vi "sequence utility.vi"(7 "sequence in":string[](array[string]), 8 "error in (no error)":errorcluster, 9 "sequence path":path=path "C:/Users/shared/Sequences/MPMS_LCR_Tsweep.vi.txt", 10 "platform":u16(ring)=1 items=["Mac", "PC"], 11 "export?":bool) -> (0 "error out":errorcluster, 2 "changed sequence":string[](array[string]), 3 "do not update seq.":bool)   [LabVIEW 2024]
doc: "Sequence Program with the Message Handling Queue (MHQ) for the National High Magnetic Field Laboratory in Tallahassee, Florida. \nOnce you understand how the programs works, you should be able to modify this program easily. If you have any questions, contact Minseong Lee(ml10k@my.fsu.edu), who first made this program in June, 2015."
panel:
  in  "edit":bool
  in  "audit":bool
  in  "accept/return":bool
  in  "Loop":bool
  in  "Replace":bool
  in  "cancel":bool
  out "Buffer Edit":string[](array[string])=["Wait for 1 s", "Wait for 2 s", "Wait for 1.1 s", "Wait for 1.2 s"]
  out "Path":path=path "C:/Users/shared/Sequences/MPMS_LCR_Tsweep.vi.txt"
  out "Buffer History":string[](array[string])
  in  "New Button":bool caption="New"
  in  "Commands":string(tree)="Wait for"
  in  "Sequence":i32[](listbox)=[4]
  in  "Save Button":bool caption="Save"
  in  "Save As Button":bool caption="Save As"
  out "Cursor Position":i32=4
  in  "Open Button":bool caption="Open"
  # "Sequence Editor"
  # "changes to the main monovu.vi"
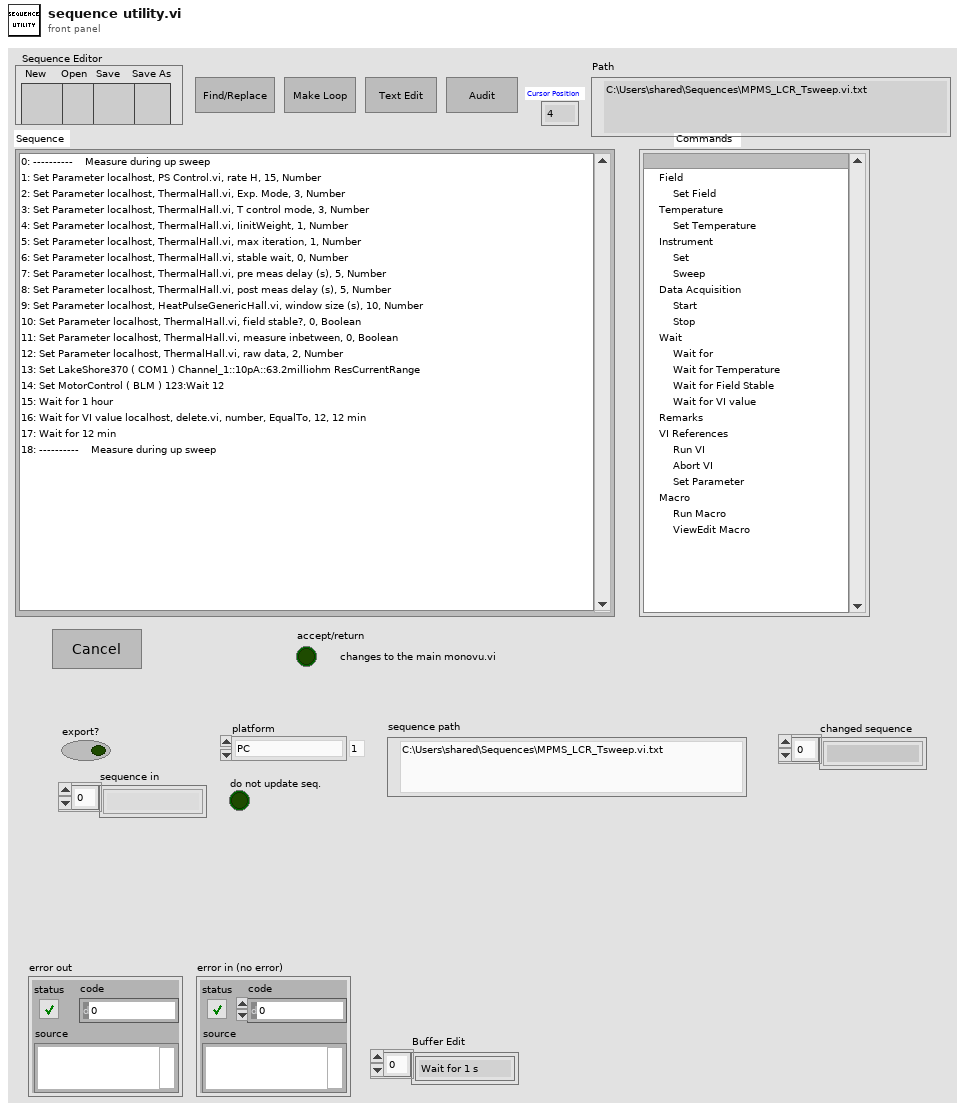
[diagram p1: front panel]
types:
  T1 = cluster{"No. of command":i32, "Parameters":string[], "Address":refnum<visa-resource-name>, "Boolean":bool, "No. of line":i32, "Initial Time":timestamp, "Current Time":timestamp, "Sequence status":string, "Sequence":refnum<vi>, "Temp_Check":i32, "Sequence_History":string, "Subsequence":string[]}
  T2 = cluster{"number of line":i32, "Signal":bool, "Command":string, "Sequence Reference":refnum<vi>, "Add or modification":bool}
  T3 = typedef "Command_Message.ctl" = cluster{"No. of command":i32, "Parameters":string[], "Address":refnum<visa-resource-name>, "Boolean":bool, "No. of line":i32, "Initial Time":timestamp, "Current Time":timestamp, "Status":string, "Sequence Ref.":refnum<vi>, "Temp check":i32, "Sequence_History":string, "Subsequence":string[]}
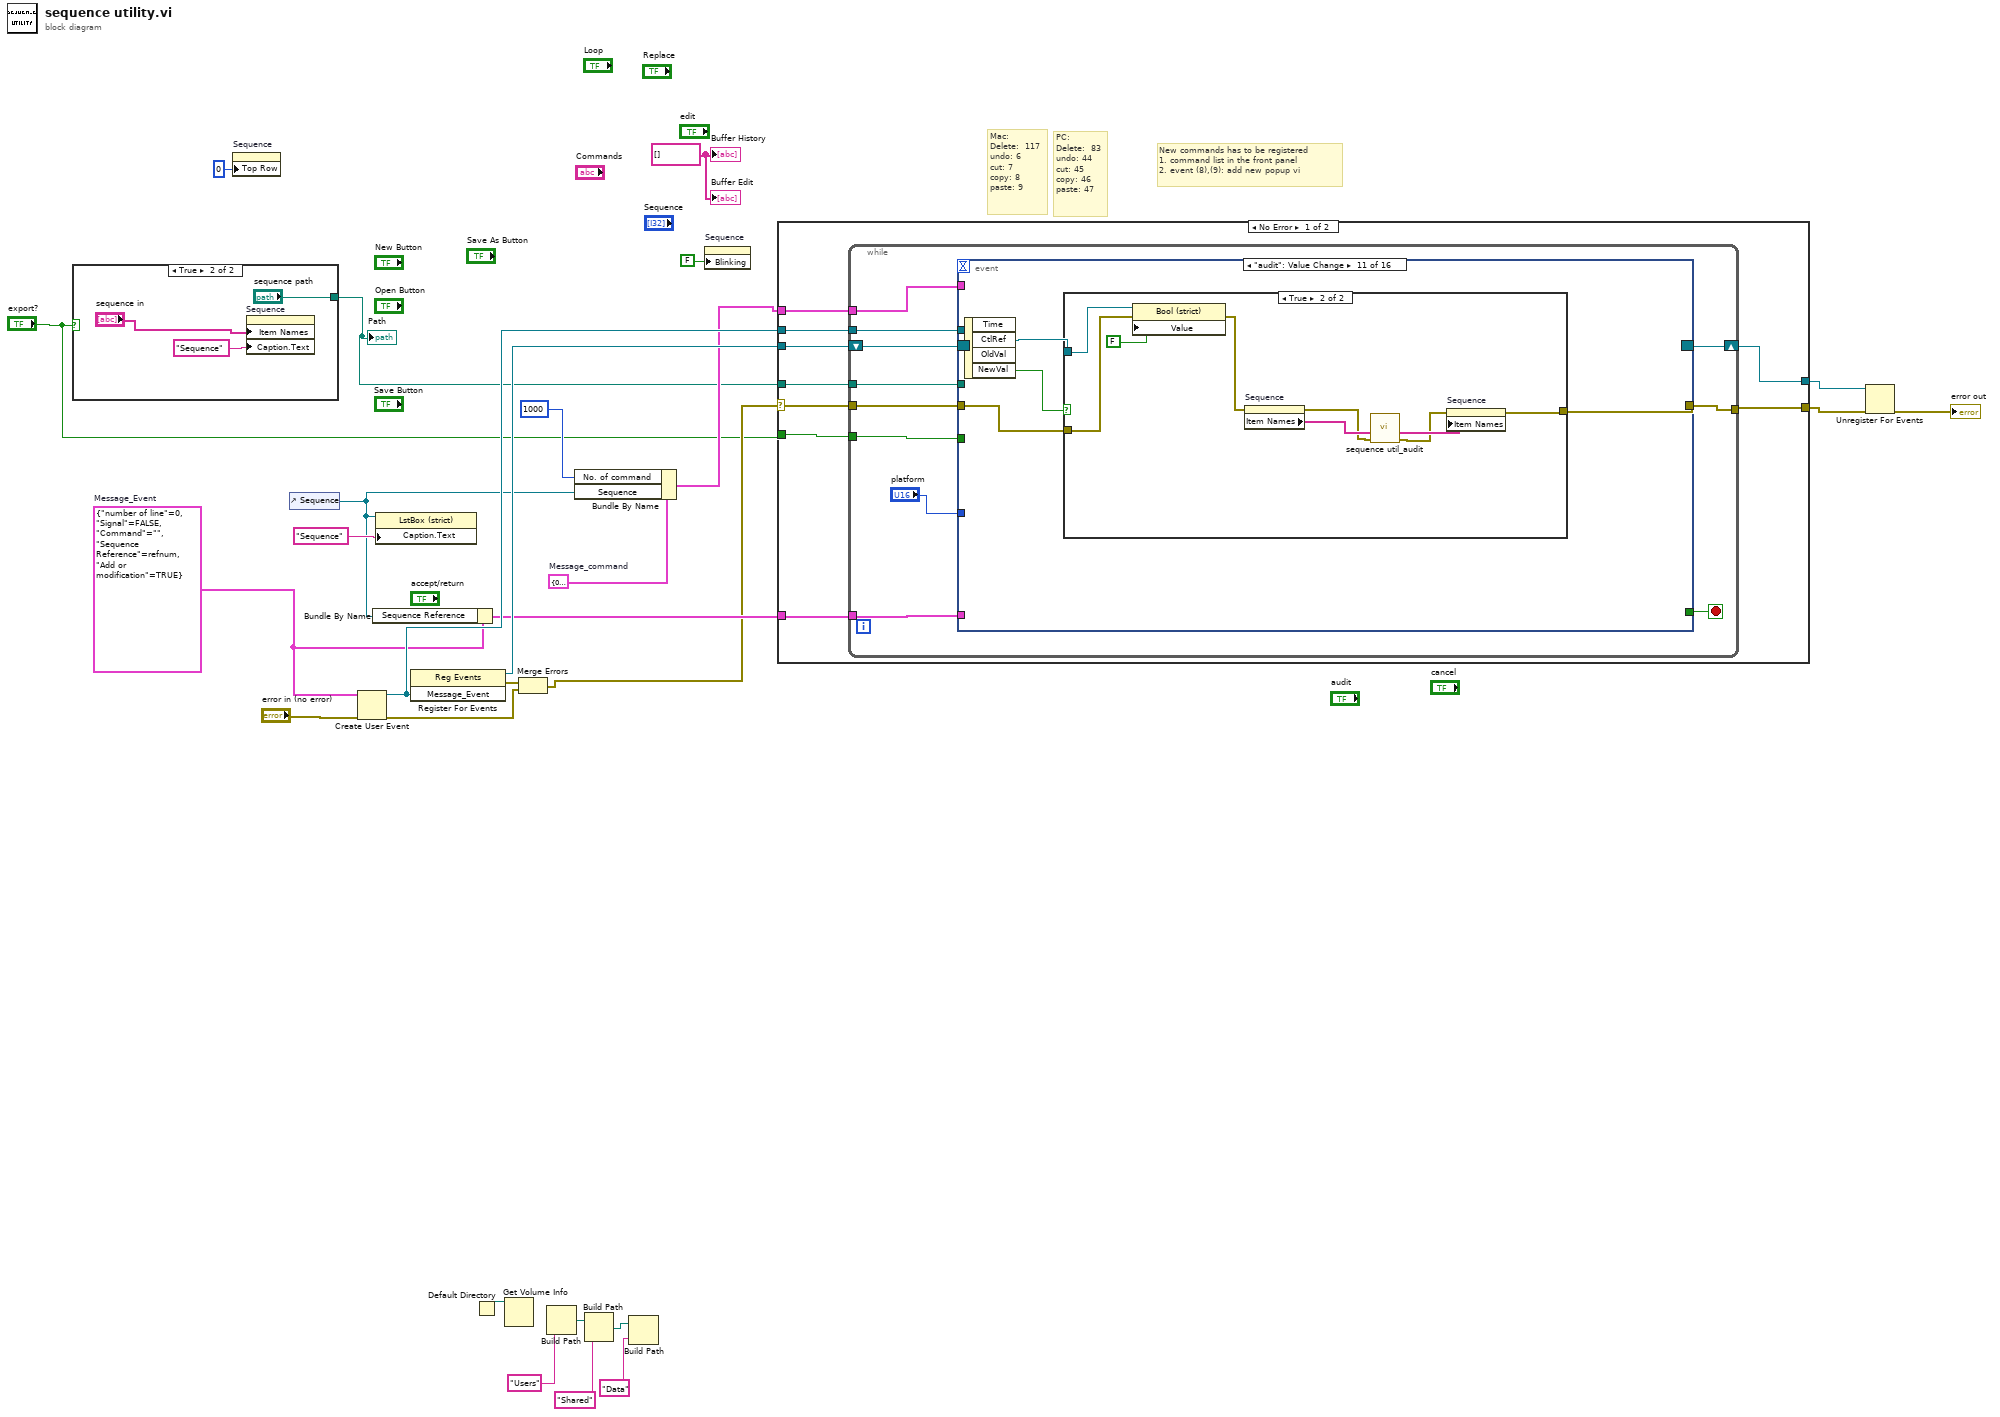
[diagram p0: block diagram]
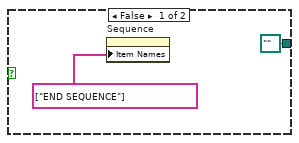
[diagram p2: hidden frame]
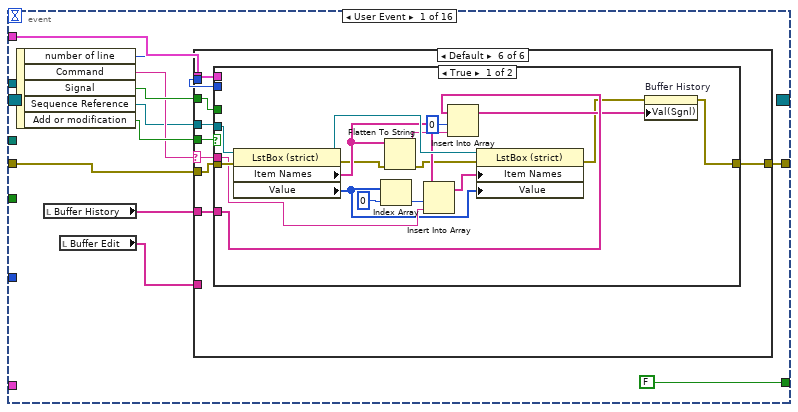
[diagram p3: hidden frame]
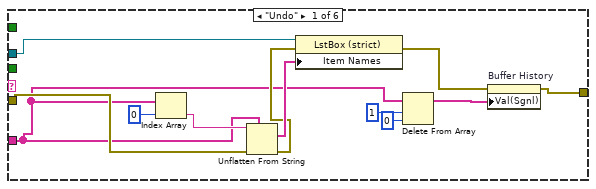
[diagram p4: hidden frame]
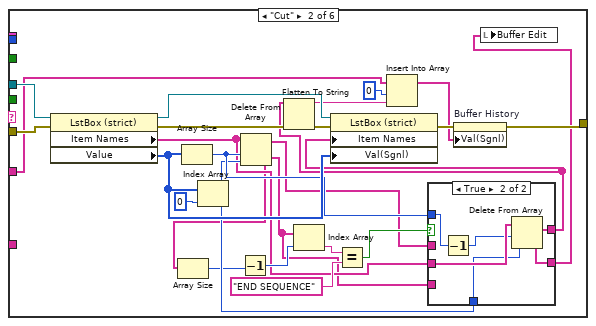
[diagram p5: hidden frame]
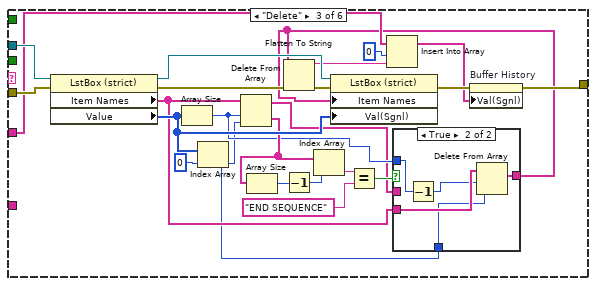
[diagram p7: hidden frame]
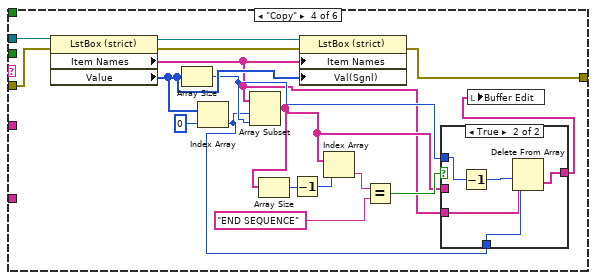
[diagram p9: hidden frame]
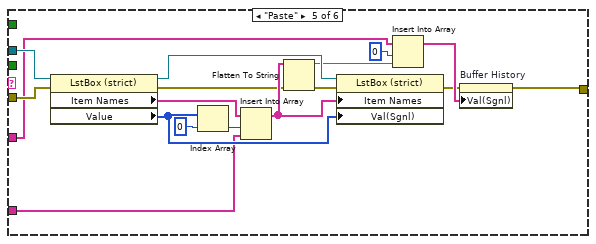
[diagram p11: hidden frame]
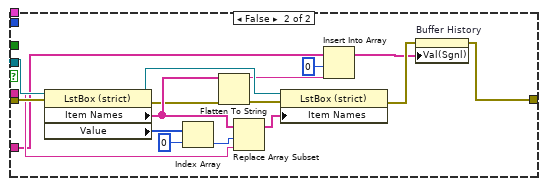
[diagram p12: hidden frame]
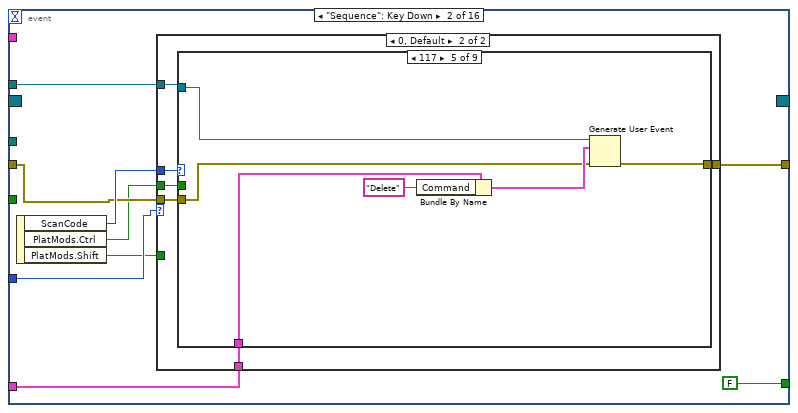
[diagram p13: hidden frame]
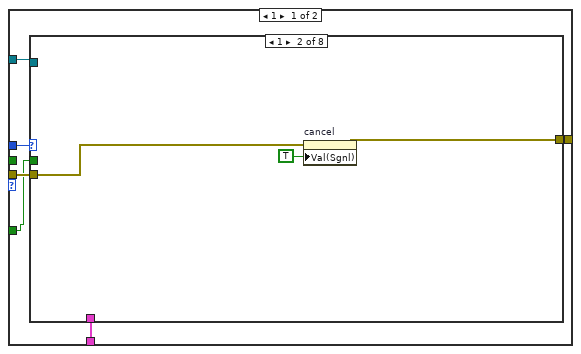
[diagram p14: hidden frame]
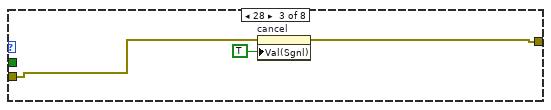
[diagram p16: hidden frame]
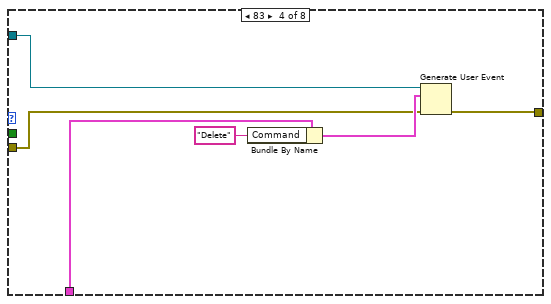
[diagram p17: hidden frame]
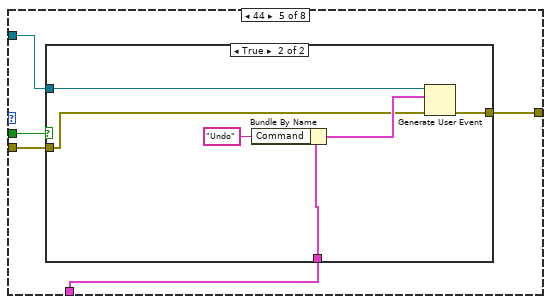
[diagram p18: hidden frame]
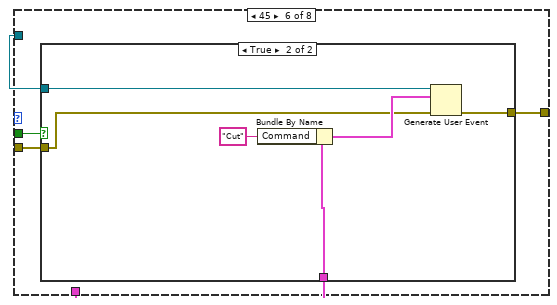
[diagram p20: hidden frame]
diagram:
  w5 = T1 {"No. of command"=0, "Parameters"=[], "Address"="", "Boolean"=TRUE, "No. of line"=0, "Initial Time"=timestamp(0 s since 1904-01-01), "Current Time"=timestamp(0 s since 1904-01-01), "Sequence status"="", "Sequence"=refnum, "Temp_Check"=0, "Sequence_History"="", "Subsequence"=[]}  # Message_command
  w15 = string[] []
  w20 = T2 {"number of line"=0, "Signal"=FALSE, "Command"="", "Sequence Reference"=refnum, "Add or modification"=TRUE}  # Message_Event
  # "New commands has to be registered\n1. command list in the front panel\n2. event (8),(9): add new popup vi"
  # "PC:\nDelete:  83\nundo: 44\ncut: 45\ncopy: 46\npaste: 47"
  # "Mac:\nDelete:  117\nundo: 6\ncut: 7\ncopy: 8\npaste: 9"
  n1 = case shown="True" "export?" {
    tunnel: [path "" ("sequence path") "sequence path"] -> w1
    frame False {
      n2 = property on="Sequence" class="LstBox (strict)"("Item Names"=string[] ["END SEQUENCE"]) -> ()  [unwired: 2 in, 2 out]
    }
    frame True {
      n3 = property on="Sequence" class="LstBox (strict)"("Item Names"="sequence in", "Caption.Text"="Sequence") -> ()  [unwired: 2 in, 2 out]
    }
  }
  "Path" <- w1
  n4 = property on="Sequence" class="LstBox (strict)"("Top Row"=0) -> ()  [unwired: 2 in, 2 out]
  n5 = control-ref of="Sequence"() -> (w16:refnum<vi>)
  n6 = Create User Event(user event datatype=w20, error in="error in (no error)") -> (user event=w23:refnum<user-event>, error out=w25:errorcluster)
  n7 = Bundle By Name(cluster=w20, "Sequence Reference"=w16) -> (w19:T2)
  n8 = property class="LstBox (strict)"(reference=w16, "Caption.Text"="Sequence") -> ()  [unwired: 1 in, 2 out]
  n9 = register-events(w23) -> (reference out=w27:refnum<event-registration>, error out=w24:errorcluster)  [unwired: 2 in]
  n10 = Default Directory() -> (w8:path)
  n11 = Get Volume Info(11:w8) -> ()  [unwired: 1 in, 6 out]
  n12 = Merge Errors(w24, w25) -> (w7:errorcluster)
  n13 = Build Path(name or relative path="Users") -> (appended path=w11:path)  [unwired: 1 in]
  n14 = Bundle By Name(cluster=w5, "No. of command"=1000, "Sequence"=w16) -> (w4:T1)
  n15 = Build Path(base path=w11, name or relative path="Shared") -> (appended path=w10:path)
  n16 = Build Path(base path=w10, name or relative path="Data") -> ()  [unwired: 1 out]
  n17 = property on="Sequence" class="LstBox (strict)"("Blinking"=FALSE) -> ()  [unwired: 2 in, 2 out]
  n18 = case shown="No Error" w7 {
    selector: w7 -> [w40 w979]
    tunnel: [w35 w979] -> w21
    tunnel: w23 -> [w39 _]
    tunnel: w27 -> [w41 w978]
    tunnel: w4 -> [w38 _]
    tunnel: [w37 w978] -> w22
    tunnel: w19 -> [w36 _]
    tunnel: w1 -> [w34 _]
    tunnel: "export?" -> [w33 _]
    frame No Error {
      n19 = while {
        tunnel: w39 -> [w50]
        tunnel: w40 -> [w49]
        tunnel: [w48] -> w35
        tunnel: w38 -> [w47]
        shift-right: [w46] -> w37
        shift-left: w41 -> [w52]
        tunnel: w36 -> [w45]
        tunnel: w34 -> [w44]
        tunnel: w33 -> [w43]
        stop <- w51 stop-if-true
        # "Event_Handler"
        n20 = event shown="[10] \"audit\": Value Change" {
          selector: w52 -> [_ _ _ _ _ _ _ _ _ _ _ _ _ _ _ _]
          dyn-events: [_ _ _ _ _ _ _ _ _ _ _ _ _ _ _ _] -> w46
          timeout: _ -> [_ _ _ _ _ _ _ _ _ _ _ _ _ _ _ _]
          tunnel: [FALSE ("NewVal") FALSE ("NewVal") FALSE ("NewVal") FALSE ("NewVal") FALSE ("NewVal") FALSE ("NewVal") FALSE ("NewVal") FALSE ("NewVal") _ _ _ _ FALSE ("NewVal") FALSE ("NewVal") FALSE ("NewVal") TRUE ("NewVal")] -> w51
          tunnel: w50 -> [_ w227 w370 _ _ _ _ _ _ _ _ _ w590 w842 _ _]
          tunnel: w49 -> [w63 w228 w372 w402 w440 w454 w482 w509 w533 w547 w561 w575 w593 w851 w967 w975]
          tunnel: [w62 w226 w371 w401 w438 w453 w481 w508 w534 w548 w562 w576 w591 w838 w967 w975] -> w48
          tunnel: w47 -> [w61 _ _ _ _ _ _ _ _ _ _ _ _ w853 _ _]
          tunnel: w45 -> [_ w229 w369 _ _ _ _ _ _ _ _ _ w589 w843 _ _]
          tunnel: w44 -> [_ _ _ _ _ _ _ _ _ _ _ _ _ _ _ _]
          tunnel: w43 -> [_ _ _ _ _ _ _ _ _ _ _ _ _ _ _ _]
          tunnel: "platform" -> [_ w223 _ _ _ _ _ _ _ _ _ _ _ _ _ _]
          event User Event {
            n21 = event-data() -> ("number of line"=w60:i32, "Command"=w55:string, "Signal"=w58:bool, "Sequence Reference"=w53:refnum<vi>, "Add or modification"=w57:bool)  [unwired: 1 in]
            n22 = local read "Buffer History"() -> (w56:string[])
            n23 = local read "Buffer Edit"() -> (w54:string[])
            n24 = case shown="Default" w55 {
              selector: w55 -> [_ _ _ _ _ w179]
              tunnel: w63 -> [w67 w99 w131 w154 w177 w187]
              tunnel: [w65 w89 w121 w149 w162 w186] -> w62
              tunnel: w61 -> [_ _ _ _ _ w185]
              tunnel: w60 -> [_ _ _ _ _ w184]
              tunnel: w58 -> [_ _ _ _ _ w183]
              tunnel: w53 -> [w64 w100 w132 w155 w178 w182]
              tunnel: w57 -> [_ _ _ _ _ w181]
              tunnel: w56 -> [w66 w94 w126 _ w168 w180]
              tunnel: w54 -> [_ _ _ _ w171 _]
              frame "Undo" {
                n25 = Index Array(array=w66, index=0) -> (element=w74:string)
                n26 = Unflatten From String(type=w66, binary string=w74, error in (no error)=w67) -> (value=w73:string[], error out=w72:errorcluster)  [unwired: 2 in, 1 out]
                n27 = property on="Property Node" class="LstBox (strict)"(reference=w64, error in=w72, "Item Names"=w73) -> (error out=w68:errorcluster)  [unwired: 1 out]
                n28 = Delete From Array(array=w66, length=1, index=0) -> (array with subset deleted=w69:string[])  [unwired: 1 out]
                n29 = property on="Buffer History" class="Arr (strict)"(error in=w68, "Val(Sgnl)"=w69) -> (error out=w65:errorcluster)  [unwired: 1 in, 1 out]
              }
              frame "Cut" {
                n30 = property on="Property Node" class="LstBox (strict)"(reference=w100, error in=w99) -> (reference out=w97:refnum<vi>, error out=w95:errorcluster, "Item Names"=w79:string[], "Value"=w96:i32[])
                n31 = Array Size(array=w96) -> (size(s)=w87:i32)
                n32 = Index Array(array=w96, index=0) -> (element=w86:i32)
                n33 = Delete From Array(array=w79, length=w87, index=w86) -> (deleted portion=w77:string[], array with subset deleted=w80:string[])
                n34 = Array Size(array=w77) -> (size(s)=w85:i32)
                n35 = Decrement(x=w85) -> (x-1=w84:i32)
                n36 = Index Array(array=w77, index=w84) -> (element=w82:string)
                n37 = Equal?(x=w82, y="END SEQUENCE") -> (x = y?=w81:bool)
                n38 = case shown="True" w81 {
                  tunnel: w79 -> [_ w108]
                  tunnel: w87 -> [_ w107]
                  tunnel: w86 -> [_ w105]
                  tunnel: [w102 w104] -> w78
                  tunnel: w80 -> [w102 _]
                  tunnel: w77 -> [w101 _]
                  tunnel: [w101 w103] -> w76
                  frame False {
                  }
                  frame True {
                    n39 = Decrement(x=w107) -> (x-1=w106:i32)
                    n40 = Delete From Array(array=w108, length=w106, index=w105) -> (deleted portion=w103:string[], array with subset deleted=w104:string[])
                  }
                }
                n41 = Flatten To String(anything=w78, error in (no error)=w95) -> (data string=w92:string, error out=w91:errorcluster)  [unwired: 2 in, 1 out]
                n42 = property on="Property Node" class="LstBox (strict)"(reference=w97, error in=w91, "Item Names"=w78, "Val(Sgnl)"=w96) -> (error out=w90:errorcluster)  [unwired: 1 out]
                n43 = Insert Into Array(array=w94, index=0, new element=w92) -> (w88:string[])
                n44 = property on="Buffer History" class="Arr (strict)"(error in=w90, "Val(Sgnl)"=w88) -> (error out=w89:errorcluster)  [unwired: 1 in, 1 out]
                n45 = local write "Buffer Edit"(w76) -> ()
              }
              frame "Delete" {
                n46 = property on="Property Node" class="LstBox (strict)"(reference=w132, error in=w131) -> (reference out=w129:refnum<vi>, error out=w127:errorcluster, "Item Names"=w113:string[], "Value"=w128:i32[])
                n47 = Array Size(array=w128) -> (size(s)=w112:i32)
                n48 = Index Array(array=w128, index=0) -> (element=w111:i32)
                n49 = Delete From Array(array=w113, length=w112, index=w111) -> (deleted portion=w119:string[], array with subset deleted=w110:string[])
                n50 = Array Size(array=w119) -> (size(s)=w115:i32)
                n51 = Decrement(x=w115) -> (x-1=w114:i32)
                n52 = Index Array(array=w119, index=w114) -> (element=w118:string)
                n53 = Equal?(x=w118, y="END SEQUENCE") -> (x = y?=w116:bool)
                n54 = case shown="True" w116 {
                  tunnel: w113 -> [_ w138]
                  tunnel: w112 -> [_ w137]
                  tunnel: w111 -> [_ w135]
                  tunnel: [w133 w134] -> w109
                  tunnel: w110 -> [w133 _]
                  frame False {
                  }
                  frame True {
                    n55 = Decrement(x=w137) -> (x-1=w136:i32)
                    n56 = Delete From Array(array=w138, length=w136, index=w135) -> (array with subset deleted=w134:string[])  [unwired: 1 out]
                  }
                }
                n57 = Flatten To String(anything=w109, error in (no error)=w127) -> (data string=w124:string, error out=w123:errorcluster)  [unwired: 2 in, 1 out]
                n58 = property on="Property Node" class="LstBox (strict)"(reference=w129, error in=w123, "Item Names"=w109, "Val(Sgnl)"=w128) -> (error out=w122:errorcluster)  [unwired: 1 out]
                n59 = Insert Into Array(array=w126, index=0, new element=w124) -> (w120:string[])
                n60 = property on="Buffer History" class="Arr (strict)"(error in=w122, "Val(Sgnl)"=w120) -> (error out=w121:errorcluster)  [unwired: 1 in, 1 out]
              }
              frame "Copy" {
                n61 = property on="Property Node" class="LstBox (strict)"(reference=w155, error in=w154) -> (reference out=w152:refnum<vi>, error out=w151:errorcluster, "Item Names"=w139:string[], "Value"=w150:i32[])
                n62 = Array Size(array=w150) -> (size(s)=w143:i32)
                n63 = Index Array(array=w150, index=0) -> (element=w142:i32)
                n64 = Array Subset(array=w139, index=w142, length=w143) -> (w141:string[])
                n65 = Array Size(array=w141) -> (size(s)=w148:i32)
                n66 = Decrement(x=w148) -> (x-1=w147:i32)
                n67 = property on="Property Node" class="LstBox (strict)"(reference=w152, error in=w151, "Item Names"=w139, "Val(Sgnl)"=w150) -> (error out=w149:errorcluster)  [unwired: 1 out]
                n68 = Index Array(array=w141, index=w147) -> (element=w146:string)
                n69 = Equal?(x=w146, y="END SEQUENCE") -> (x = y?=w144:bool)
                n70 = case shown="True" w144 {
                  tunnel: w143 -> [_ w161]
                  tunnel: w142 -> [_ w159]
                  tunnel: [w156 w157] -> w140
                  tunnel: w141 -> [w156 _]
                  tunnel: w139 -> [_ w158]
                  frame False {
                  }
                  frame True {
                    n71 = Decrement(x=w161) -> (x-1=w160:i32)
                    n72 = Delete From Array(array=w158, length=w160, index=w159) -> (deleted portion=w157:string[])  [unwired: 1 out]
                  }
                }
                n73 = local write "Buffer Edit"(w140) -> ()
              }
              frame "Paste" {
                n74 = property on="Property Node" class="LstBox (strict)"(reference=w178, error in=w177) -> (reference out=w175:refnum<vi>, error out=w165:errorcluster, "Item Names"=w172:string[], "Value"=w174:i32[])
                n75 = Index Array(array=w174, index=0) -> (element=w173:i32)
                n76 = Insert Into Array(array=w172, index=w173, new element=w171) -> (w169:string[])
                n77 = Flatten To String(anything=w169, error in (no error)=w165) -> (data string=w170:string, error out=w164:errorcluster)  [unwired: 2 in, 1 out]
                n78 = property on="Property Node" class="LstBox (strict)"(reference=w175, error in=w164, "Item Names"=w169, "Val(Sgnl)"=w174) -> (error out=w163:errorcluster)  [unwired: 1 out]
                n79 = Insert Into Array(array=w168, index=0, new element=w170) -> (w166:string[])
                n80 = property on="Buffer History" class="Arr (strict)"(error in=w163, "Val(Sgnl)"=w166) -> (error out=w162:errorcluster)  [unwired: 1 in, 1 out]
              }
              frame Default {
                n81 = case shown="True" w181 {
                  tunnel: w187 -> [w204 w221]
                  tunnel: [w188 w205] -> w186
                  tunnel: w185 -> [_ _]
                  tunnel: w184 -> [_ _]
                  tunnel: w183 -> [_ _]
                  tunnel: w182 -> [w203 w220]
                  tunnel: w179 -> [w202 w219]
                  tunnel: w180 -> [w201 w218]
                  frame True {
                    n82 = property class="LstBox (strict)"(reference=w203, error in=w204) -> (reference out=w198:refnum<vi>, error out=w192:errorcluster, "Item Names"=w194:string[], "Value"=w197:i32[])
                    n83 = Index Array(array=w197, index=0) -> (element=w199:i32)
                    n84 = Flatten To String(anything=w194, error in (no error)=w192) -> (data string=w195:string, error out=w193:errorcluster)  [unwired: 2 in, 1 out]
                    n85 = Insert Into Array(array=w194, index=w199, new element=w202) -> (w196:string[])
                    n86 = Insert Into Array(array=w201, index=0, new element=w195) -> (w190:string[])
                    n87 = property class="LstBox (strict)"(reference=w198, error in=w193, "Item Names"=w196, "Value"=w197) -> (error out=w189:errorcluster)  [unwired: 1 out]
                    n88 = property on="Buffer History" class="Arr (strict)"(error in=w189, "Val(Sgnl)"=w190) -> (error out=w188:errorcluster)  [unwired: 1 in, 1 out]
                  }
                  frame False {
                    n89 = property class="LstBox (strict)"(reference=w220, error in=w221) -> (reference out=w215:refnum<vi>, error out=w210:errorcluster, "Item Names"=w211:string[], "Value"=w214:i32[])
                    n90 = Index Array(array=w214, index=0) -> (element=w216:i32)
                    n91 = Flatten To String(anything=w211, error in (no error)=w210) -> (data string=w213:string, error out=w209:errorcluster)  [unwired: 2 in, 1 out]
                    n92 = Replace Array Subset(array=w211, new element=w219, index=w216) -> (w212:string[])
                    n93 = property class="LstBox (strict)"(reference=w215, error in=w209, "Item Names"=w212) -> (error out=w207:errorcluster)  [unwired: 1 out]
                    n94 = Insert Into Array(array=w218, index=0, new element=w213) -> (w206:string[])
                    n95 = property on="Buffer History" class="Arr (strict)"(error in=w207, "Val(Sgnl)"=w206) -> (error out=w205:errorcluster)  [unwired: 1 in, 1 out]
                  }
                }
              }
            }
          }
          event "Sequence": Key Down {
            n96 = event-data() -> ("ScanCode"=w230:i16, "PlatMods.Ctrl"=w224:bool, "PlatMods.Shift"=w222:bool)  [unwired: 1 in]
            n97 = case shown="0, Default" w223 {
              tunnel: w230 -> [w236 w303]
              tunnel: w229 -> [w235 w302]
              tunnel: w228 -> [w234 w301]
              tunnel: w227 -> [w233 w300]
              tunnel: [w232 w299] -> w226
              tunnel: w224 -> [_ w298]
              tunnel: w222 -> [w231 _]
              frame 1 {
                n98 = case shown="1" w236 {
                  tunnel: w235 -> [_ _ _ w248 w251 w263 w275 w287]
                  tunnel: w234 -> [w237 w239 w243 w246 w253 w265 w277 w289]
                  tunnel: w233 -> [_ _ _ w245 w250 w262 w274 w286]
                  tunnel: [w237 w240 w242 w244 w252 w264 w276 w288] -> w232
                  tunnel: w231 -> [_ _ _ _ w254 w266 w278 w290]
                  frame 0, Default {
                  }
                  frame 1 {
                    n99 = property on="cancel" class="Bool (strict)"(error in=w239, "Val(Sgnl)"=TRUE ("Value (Signaling)")) -> (error out=w240:errorcluster)  [unwired: 1 in, 1 out]
                  }
                  frame 28 {
                    n100 = property on="cancel" class="Bool (strict)"(error in=w243, "Val(Sgnl)"=TRUE ("Value (Signaling)")) -> (error out=w242:errorcluster)  [unwired: 1 in, 1 out]
                  }
                  frame 83 {
                    n101 = Bundle By Name(cluster=w248, "Command"="Delete") -> (w247:T2)
                    n102 = Generate User Event(user event=w245, event data cluster=w247, error in=w246) -> (error out=w244:errorcluster)  [unwired: 1 in, 1 out]
                  }
                  frame 44 {
                    n103 = case shown="True" w254 {
                      tunnel: w253 -> [w255 w257]
                      tunnel: [w255 w259] -> w252
                      tunnel: w251 -> [_ w258]
                      tunnel: w250 -> [_ w256]
                      frame False {
                      }
                      frame True {
                        n104 = Bundle By Name(cluster=w258, "Command"="Undo") -> (w260:T2)
                        n105 = Generate User Event(user event=w256, event data cluster=w260, error in=w257) -> (error out=w259:errorcluster)  [unwired: 1 in, 1 out]
                      }
                    }
                  }
                  frame 45 {
                    n106 = case shown="True" w266 {
                      tunnel: w265 -> [w267 w269]
                      tunnel: [w267 w271] -> w264
                      tunnel: w263 -> [_ w270]
                      tunnel: w262 -> [_ w268]
                      frame False {
                      }
                      frame True {
                        n107 = Bundle By Name(cluster=w270, "Command"="Cut") -> (w272:T2)
                        n108 = Generate User Event(user event=w268, event data cluster=w272, error in=w269) -> (error out=w271:errorcluster)  [unwired: 1 in, 1 out]
                      }
                    }
                  }
                  frame 46 {
                    n109 = case shown="True" w278 {
                      tunnel: w277 -> [w279 w281]
                      tunnel: [w279 w283] -> w276
                      tunnel: w275 -> [_ w282]
                      tunnel: w274 -> [_ w280]
                      frame False {
                      }
                      frame True {
                        n110 = Bundle By Name(cluster=w282, "Command"="Copy") -> (w284:T2)
                        n111 = Generate User Event(user event=w280, event data cluster=w284, error in=w281) -> (error out=w283:errorcluster)  [unwired: 1 in, 1 out]
                      }
                    }
                  }
                  frame 47 {
                    n112 = case shown="True" w290 {
                      tunnel: w289 -> [w291 w293]
                      tunnel: [w291 w295] -> w288
                      tunnel: w287 -> [_ w294]
                      tunnel: w286 -> [_ w292]
                      frame False {
                      }
                      frame True {
                        n113 = Bundle By Name(cluster=w294, "Command"="Paste") -> (w296:T2)
                        n114 = Generate User Event(user event=w292, event data cluster=w296, error in=w293) -> (error out=w295:errorcluster)  [unwired: 1 in, 1 out]
                      }
                    }
                  }
                }
              }
              frame 0, Default {
                n115 = case shown="117" w303 {
                  tunnel: w302 -> [_ _ _ _ w318 w321 w333 w345 w357]
                  tunnel: w301 -> [w304 w305 w309 w312 w316 w323 w335 w347 w359]
                  tunnel: w300 -> [_ _ _ _ w315 w320 w332 w344 w356]
                  tunnel: [w304 w306 w308 w311 w314 w322 w334 w346 w358] -> w299
                  tunnel: w298 -> [_ _ _ _ _ w324 w336 w348 w360]
                  frame 0, Default {
                  }
                  frame 36 {
                    n116 = property on="cancel" class="Bool (strict)"(error in=w305, "Val(Sgnl)"=TRUE ("Value (Signaling)")) -> (error out=w306:errorcluster)  [unwired: 1 in, 1 out]
                  }
                  frame 76 {
                    n117 = property on="cancel" class="Bool (strict)"(error in=w309, "Val(Sgnl)"=TRUE ("Value (Signaling)")) -> (error out=w308:errorcluster)  [unwired: 1 in, 1 out]
                  }
                  frame 53 {
                    n118 = property on="cancel" class="Bool (strict)"(error in=w312, "Val(Sgnl)"=TRUE ("Value (Signaling)")) -> (error out=w311:errorcluster)  [unwired: 1 in, 1 out]
                  }
                  frame 117 {
                    n119 = Bundle By Name(cluster=w318, "Command"="Delete") -> (w317:T2)
                    n120 = Generate User Event(user event=w315, event data cluster=w317, error in=w316) -> (error out=w314:errorcluster)  [unwired: 1 in, 1 out]
                  }
                  frame 6 {
                    n121 = case shown="True" w324 {
                      tunnel: w323 -> [w325 w327]
                      tunnel: [w325 w329] -> w322
                      tunnel: w321 -> [_ w328]
                      tunnel: w320 -> [_ w326]
                      frame False {
                      }
                      frame True {
                        n122 = Bundle By Name(cluster=w328, "Command"="Undo") -> (w330:T2)
                        n123 = Generate User Event(user event=w326, event data cluster=w330, error in=w327) -> (error out=w329:errorcluster)  [unwired: 1 in, 1 out]
                      }
                    }
                  }
                  frame 7 {
                    n124 = case shown="True" w336 {
                      tunnel: w335 -> [w337 w339]
                      tunnel: [w337 w341] -> w334
                      tunnel: w333 -> [_ w340]
                      tunnel: w332 -> [_ w338]
                      frame False {
                      }
                      frame True {
                        n125 = Bundle By Name(cluster=w340, "Command"="Cut") -> (w342:T2)
                        n126 = Generate User Event(user event=w338, event data cluster=w342, error in=w339) -> (error out=w341:errorcluster)  [unwired: 1 in, 1 out]
                      }
                    }
                  }
                  frame 8 {
                    n127 = case shown="True" w348 {
                      tunnel: w347 -> [w349 w351]
                      tunnel: [w349 w353] -> w346
                      tunnel: w345 -> [_ w352]
                      tunnel: w344 -> [_ w350]
                      frame False {
                      }
                      frame True {
                        n128 = Bundle By Name(cluster=w352, "Command"="Copy") -> (w354:T2)
                        n129 = Generate User Event(user event=w350, event data cluster=w354, error in=w351) -> (error out=w353:errorcluster)  [unwired: 1 in, 1 out]
                      }
                    }
                  }
                  frame 9 {
                    n130 = case shown="True" w360 {
                      tunnel: w359 -> [w361 w363]
                      tunnel: [w361 w365] -> w358
                      tunnel: w357 -> [_ w364]
                      tunnel: w356 -> [_ w362]
                      frame False {
                      }
                      frame True {
                        n131 = Bundle By Name(cluster=w364, "Command"="Paste") -> (w366:T2)
                        n132 = Generate User Event(user event=w362, event data cluster=w366, error in=w363) -> (error out=w365:errorcluster)  [unwired: 1 in, 1 out]
                      }
                    }
                  }
                }
              }
            }
          }
          event "Sequence": Shortcut Menu Selection (User) {
            n133 = event-data() -> ("ItemTag"=w373:string)  [unwired: 1 in]
            n134 = case shown="\"Cut\"" w373 {
              selector: w373 -> [_ w378 w384 w390 w396]
              tunnel: w372 -> [w374 w376 w382 w388 w394]
              tunnel: [w374 w375 w381 w387 w393] -> w371
              tunnel: w370 -> [_ w380 w386 w392 w398]
              tunnel: w369 -> [_ w379 w385 w391 w397]
              frame Default {
              }
              frame "Undo" {
                n135 = Bundle By Name(cluster=w379, "Command"=w378) -> (w377:T2)
                n136 = Generate User Event(user event=w380, event data cluster=w377, error in=w376) -> (error out=w375:errorcluster)  [unwired: 1 in, 1 out]
              }
              frame "Cut" {
                n137 = Bundle By Name(cluster=w385, "Command"=w384) -> (w383:T2)
                n138 = Generate User Event(user event=w386, event data cluster=w383, error in=w382) -> (error out=w381:errorcluster)  [unwired: 1 in, 1 out]
              }
              frame "Copy" {
                n139 = Bundle By Name(cluster=w391, "Command"=w390) -> (w389:T2)
                n140 = Generate User Event(user event=w392, event data cluster=w389, error in=w388) -> (error out=w387:errorcluster)  [unwired: 1 in, 1 out]
              }
              frame "Paste" {
                n141 = Bundle By Name(cluster=w397, "Command"=w396) -> (w395:T2)
                n142 = Generate User Event(user event=w398, event data cluster=w395, error in=w394) -> (error out=w393:errorcluster)  [unwired: 1 in, 1 out]
              }
            }
          }
          event "New Button": Value Change {
            n143 = event-data() -> ("NewVal"=w403:bool, "CtlRef"=w400:refnum<vi>)  [unwired: 1 in]
            n144 = case shown="True" w403 {
              tunnel: w402 -> [w404 w420]
              tunnel: [w404 w412] -> w401
              tunnel: w400 -> [_ w415]
              frame False {
              }
              frame True {
                n145 = property on="Sequence" class="LstBox (strict)"(error in=w420) -> (error out=w411:errorcluster, "Caption.Text"=w419:string, "Item Names"=w416:string[])  [unwired: 1 in, 1 out]
                n146 = property on="Buffer History" class="Arr (strict)"(error in=w411) -> (error out=w410:errorcluster, "Value"=w409:string[])  [unwired: 1 in, 1 out]
                n147 = Equal?(x=w419, y="Sequence*") -> (x = y?=w417:bool)
                n148 = case shown="False" w417 {
                  tunnel: w410 -> [w425 w436]
                  tunnel: w416 -> [_ w437]
                  tunnel: [w426 w431] -> w408
                  tunnel: w415 -> [w424 w430]
                  tunnel: [w424 w430] -> w414
                  tunnel: w409 -> [_ w428]
                  tunnel: [string[] [] ("Buffer out") w427] -> w406
                  frame False {
                    n149 = property on="Sequence" class="LstBox (strict)"(error in=w425, "Item Names"=string[] ["END SEQUENCE"], "Caption.Text"="Sequence") -> (error out=w426:errorcluster)  [unwired: 1 in, 1 out]
                  }
                  frame True {
                    n150 = property on="Path" class="Path"(error in=w436) -> (error out=w435:errorcluster, "Value"=w434:path)  [unwired: 1 in, 1 out]
                    n151 = call "New_File.vi"("error in (no error)"=w435, "Path"=w434, "Buffer in"=w428, "Sequence in"=w437) -> ("error out"=w433:errorcluster, "Sequence Caption"=w429:string, "Buffer out"=w427:string[], "Sequence_out"=w432:string[])  [unwired: 4 in]
                    n152 = property on="Sequence" class="LstBox (strict)"(error in=w433, "Item Names"=w432, "Caption.Text"=w429) -> (error out=w431:errorcluster)  [unwired: 1 in, 1 out]
                  }
                }
                n153 = property on="Buffer History" class="Arr (strict)"(error in=w408, "Value"=w406) -> (error out=w407:errorcluster)  [unwired: 1 in, 1 out]
                n154 = property class="Bool (strict)"(reference=w414, error in=w407, "Value"=FALSE) -> (error out=w412:errorcluster)  [unwired: 1 out]
                n155 = property on="Sequence" class="LstBox (strict)"("Top Row"=0) -> ()  [unwired: 2 in, 2 out]
              }
            }
          }
          event "Buffer History": Value Change {
            n156 = event-data() -> ("NewVal"=w444:string[])  [unwired: 1 in]
            n157 = Array Size(array=w444) -> (size(s)=w443:i32)
            n158 = Equal?(x=w443, y=0) -> (x = y?=w441:bool)
            n159 = case shown="False" w441 {
              tunnel: w440 -> [w446 w449]
              tunnel: [w445 w448] -> w438
              frame True {
                n160 = property on="Sequence" class="LstBox (strict)"(error in=w446, "Caption.Text"="Sequence") -> (error out=w445:errorcluster)  [unwired: 1 in, 1 out]
              }
              frame False {
                n161 = property on="Sequence" class="LstBox (strict)"(error in=w449, "Caption.Text"="Sequence*") -> (error out=w448:errorcluster)  [unwired: 1 in, 1 out]
              }
            }
          }
          event "Open Button": Value Change {
            n162 = event-data() -> ("NewVal"=w455:bool, "CtlRef"=w452:refnum<vi>)  [unwired: 1 in]
            n163 = case shown="True" w455 {
              tunnel: w454 -> [w456 w478]
              tunnel: [w456 w459] -> w453
              tunnel: w452 -> [_ w462]
              frame False {
              }
              frame True {
                n164 = property on="Sequence" class="LstBox (strict)"(error in=w478) -> (error out=w474:errorcluster, "Caption.Text"=w476:string, "Item Names"=w475:string[])  [unwired: 1 in, 1 out]
                n165 = Equal?(x=w476, y="Sequence*") -> (x = y?=w463:bool)
                n166 = property on="Buffer History" class="Arr (strict)"(error in=w474) -> (error out=w472:errorcluster, "Value"=w473:string[])  [unwired: 1 in, 1 out]
                n167 = property on="Path" class="Path"(error in=w472) -> (error out=w470:errorcluster, "Value"=w471:path)  [unwired: 1 in, 1 out]
                n168 = call "Open_File.vi"("Message?"=w463, "Path in"=w471, "error in (no error)"=w470, "Sequence in"=w475, "Buffer in"=w473, "Sequence Caption in"=w476) -> ("error out"=w458:errorcluster, "Sequence out"=w468:string[], "Buffer out"=w466:string[], "Sequence Caption out"=w469:string, "Path out"=w464:path, "top row"=w457:i32)
                n169 = property on="Sequence" class="LstBox (strict)"("Top Row"=w457) -> ()  [unwired: 2 in, 2 out]
                n170 = property on="Sequence" class="LstBox (strict)"(error in=w458, "Item Names"=w468, "Caption.Text"=w469) -> (error out=w467:errorcluster)  [unwired: 1 in, 1 out]
                n171 = property on="Buffer History" class="Arr (strict)"(error in=w467, "Value"=w466) -> (error out=w465:errorcluster)  [unwired: 1 in, 1 out]
                n172 = property on="Path" class="Path"(error in=w465, "Value"=w464) -> (error out=w461:errorcluster)  [unwired: 1 in, 1 out]
                n173 = property class="Bool (strict)"(reference=w462, error in=w461, "Value"=FALSE) -> (error out=w459:errorcluster)  [unwired: 1 out]
              }
            }
          }
          event "Save Button": Value Change {
            n174 = event-data() -> ("NewVal"=w483:bool, "CtlRef"=w480:refnum<vi>)  [unwired: 1 in]
            n175 = case shown="True" w483 {
              tunnel: w482 -> [w484 w501]
              tunnel: [w484 w485] -> w481
              tunnel: w480 -> [_ w488]
              frame False {
              }
              frame True {
                n176 = property on="Path" class="Path"(error in=w501) -> (error out=w500:errorcluster, "Value"=w503:path)  [unwired: 1 in, 1 out]
                n177 = Not Equal?(x=path "", y=w503) -> (x != y?=w504:bool)
                n178 = property on="Buffer History" class="Arr (strict)"(error in=w500) -> (error out=w499:errorcluster, "Value"=w502:string[])  [unwired: 1 in, 1 out]
                n179 = property on="Sequence" class="LstBox (strict)"(error in=w499) -> (error out=w498:errorcluster, "Item Names"=w497:string[], "Caption.Text"=w496:string)  [unwired: 1 in, 1 out]
                n180 = call "Save_File.vi"("Sequence caption in"=w496, "Path?"=w504, "error in (no error)"=w498, "Sequence in"=w497, "Buffer in"=w502, "Path in"=w503) -> ("error out"=w495:errorcluster, "Sequence out"=w491:string[], "Buffer out"=w493:string[], "Path out"=w489:path, "Sequence caption out"=w492:string)  [unwired: 1 in]
                n181 = property on="Buffer History" class="Arr (strict)"(error in=w495, "Value"=w493) -> (error out=w494:errorcluster)  [unwired: 1 in, 1 out]
                n182 = property on="Sequence" class="LstBox (strict)"(error in=w494, "Item Names"=w491, "Caption.Text"=w492) -> (error out=w490:errorcluster)  [unwired: 1 in, 1 out]
                n183 = property on="Path" class="Path"(error in=w490, "Value"=w489) -> (error out=w487:errorcluster)  [unwired: 1 in, 1 out]
                n184 = property class="Bool (strict)"(reference=w488, error in=w487, "Value"=FALSE) -> (error out=w485:errorcluster)  [unwired: 1 out]
              }
            }
          }
          event "Save As Button": Value Change {
            n185 = event-data() -> ("NewVal"=w510:bool, "CtlRef"=w507:refnum<vi>)  [unwired: 1 in]
            n186 = case shown="True" w510 {
              tunnel: w509 -> [w511 w529]
              tunnel: [w511 w513] -> w508
              tunnel: w507 -> [_ w516]
              frame False {
              }
              frame True {
                n187 = property on="Path" class="Path"(error in=w529) -> (error out=w528:errorcluster, "Value"=w531:path)  [unwired: 1 in, 1 out]
                n188 = property on="Buffer History" class="Arr (strict)"(error in=w528) -> (error out=w527:errorcluster, "Value"=w530:string[])  [unwired: 1 in, 1 out]
                n189 = property on="Sequence" class="LstBox (strict)"(error in=w527) -> (error out=w526:errorcluster, "Item Names"=w525:string[], "Caption.Text"=w524:string)  [unwired: 1 in, 1 out]
                n190 = call "Save_File.vi"("Sequence caption in"=w524, "Path?"=FALSE, "error in (no error)"=w526, "Sequence in"=w525, "Buffer in"=w530, "Path in"=w531) -> ("error out"=w523:errorcluster, "Sequence out"=w519:string[], "Buffer out"=w521:string[], "Path out"=w517:path, "Sequence caption out"=w520:string)  [unwired: 1 in]
                n191 = property on="Buffer History" class="Arr (strict)"(error in=w523, "Value"=w521) -> (error out=w522:errorcluster)  [unwired: 1 in, 1 out]
                n192 = property on="Sequence" class="LstBox (strict)"(error in=w522, "Item Names"=w519, "Caption.Text"=w520) -> (error out=w518:errorcluster)  [unwired: 1 in, 1 out]
                n193 = property on="Path" class="Path"(error in=w518, "Value"=w517) -> (error out=w515:errorcluster)  [unwired: 1 in, 1 out]
                n194 = property class="Bool (strict)"(reference=w516, error in=w515, "Value"=FALSE) -> (error out=w513:errorcluster)  [unwired: 1 out]
              }
            }
          }
          event "Replace": Value Change {
            n195 = event-data() -> ("CtlRef"=w532:refnum<vi>, "NewVal"=w535:bool)  [unwired: 1 in, 2 out]
            n196 = case shown="True" w535 {
              tunnel: [w536 w537] -> w534
              tunnel: w533 -> [w536 w541]
              tunnel: w532 -> [_ w544]
              frame False {
              }
              frame True {
                n197 = property class="Bool (strict)"(reference=w544, error in=w541, "Value"=FALSE) -> (error out=w540:errorcluster)  [unwired: 1 out]
                n198 = property on="Sequence" class="LstBox (strict)"(error in=w540) -> (error out=w539:errorcluster, "Item Names"=w543:string[])  [unwired: 1 in, 1 out]
                n199 = call "sequence util_findNreplace.vi"("error in"=w539, "Item Names IN"=w543) -> ("error out"=w538:errorcluster, "Item Names out"=w542:string[])  [unwired: 7 in, 1 out]
                n200 = property on="Sequence" class="LstBox (strict)"(error in=w538, "Item Names"=w542) -> (error out=w537:errorcluster)  [unwired: 1 in, 1 out]
              }
            }
          }
          event "Loop": Value Change {
            n201 = event-data() -> ("CtlRef"=w546:refnum<vi>, "NewVal"=w549:bool)  [unwired: 1 in, 2 out]
            n202 = case shown="True" w549 {
              tunnel: [w550 w551] -> w548
              tunnel: w547 -> [w550 w555]
              tunnel: w546 -> [_ w558]
              frame False {
              }
              frame True {
                n203 = property class="Bool (strict)"(reference=w558, error in=w555, "Value"=FALSE) -> (error out=w554:errorcluster)  [unwired: 1 out]
                n204 = property on="Sequence" class="LstBox (strict)"(error in=w554) -> (error out=w553:errorcluster, "Item Names"=w557:string[])  [unwired: 1 in, 1 out]
                n205 = call "sequence util_makeloop.vi"("error in"=w553, "Item Names IN"=w557) -> ("error out"=w552:errorcluster, "Item Names out"=w556:string[])  [unwired: 6 in, 2 out]
                n206 = property on="Sequence" class="LstBox (strict)"(error in=w552, "Item Names"=w556) -> (error out=w551:errorcluster)  [unwired: 1 in, 1 out]
              }
            }
          }
          event "audit": Value Change {
            n207 = event-data() -> ("CtlRef"=w560:refnum<vi>, "NewVal"=w563:bool)  [unwired: 1 in, 2 out]
            n208 = case shown="True" w563 {
              tunnel: [w564 w565] -> w562
              tunnel: w561 -> [w564 w569]
              tunnel: w560 -> [_ w572]
              frame False {
              }
              frame True {
                n209 = property class="Bool (strict)"(reference=w572, error in=w569, "Value"=FALSE) -> (error out=w568:errorcluster)  [unwired: 1 out]
                n210 = property on="Sequence" class="LstBox (strict)"(error in=w568) -> (error out=w567:errorcluster, "Item Names"=w571:string[])  [unwired: 1 in, 1 out]
                n211 = call "sequence util_audit.vi"("error in"=w567, "Item Names IN"=w571) -> ("error out"=w566:errorcluster, "Item Names out"=w570:string[])  [unwired: 8 in]
                n212 = property on="Sequence" class="LstBox (strict)"(error in=w566, "Item Names"=w570) -> (error out=w565:errorcluster)  [unwired: 1 in, 1 out]
              }
            }
          }
          event "edit": Value Change {
            n213 = event-data() -> ("CtlRef"=w574:refnum<vi>, "NewVal"=w577:bool)  [unwired: 1 in, 2 out]
            n214 = case shown="True" w577 {
              tunnel: [w578 w579] -> w576
              tunnel: w575 -> [w578 w583]
              tunnel: w574 -> [_ w586]
              frame False {
              }
              frame True {
                n215 = property class="Bool (strict)"(reference=w586, error in=w583, "Value"=FALSE) -> (error out=w582:errorcluster)  [unwired: 1 out]
                n216 = property on="Sequence" class="LstBox (strict)"(error in=w582) -> (error out=w581:errorcluster, "Item Names"=w585:string[])  [unwired: 1 in, 1 out]
                n217 = call "sequence util_edit.vi"("error in"=w581, "Sequence Array"=w585) -> ("error out"=w580:errorcluster, "Item Names out"=w584:string[])  [unwired: 8 in]
                n218 = property on="Sequence" class="LstBox (strict)"(error in=w580, "Item Names"=w584) -> (error out=w579:errorcluster)  [unwired: 1 in, 1 out]
              }
            }
          }
          event "Commands": Double Click {
            n219 = event-data() -> ("Tag"=w592:string)  [unwired: 1 in]
            n220 = case shown="\"Write to VISA instrument\"" w592 {
              tunnel: w593 -> [w594 w597 w611 w625 w639 w653 w667 w681 w695 w709 w723 w737 w751 w765 w778 w792 w807 w822]
              tunnel: [w594 w599 w613 w627 w641 w655 w669 w683 w697 w711 w725 w739 w753 w767 w782 w796 w810 w825] -> w591
              tunnel: w590 -> [_ w603 w617 w631 w645 w659 w673 w687 w701 w715 w729 w743 w757 w771 w784 w797 w811 w826]
              tunnel: w589 -> [_ w598 w612 w626 w640 w654 w668 w682 w696 w710 w724 w738 w752 w766 w781 w795 w809 w824]
              frame Default {
              }
              frame "Set Field" {
                n221 = call "SetField_popup.vi"("error in (no error)"=w597) -> ("Output Line command"=w601:string, "Cancel"=w595:bool, "error out"=w602:errorcluster)  [unwired: 5 in]
                n222 = Bundle By Name(cluster=w598, "Signal"=w595, "Command"=w601, "Add or modification"=TRUE) -> (w600:T2)
                n223 = case shown="True" w595 {
                  tunnel: w603 -> [w607 _]
                  tunnel: w602 -> [w606 w608]
                  tunnel: w600 -> [w605 _]
                  tunnel: [w604 w608] -> w599
                  frame False {
                    n224 = Generate User Event(user event=w607, event data cluster=w605, error in=w606) -> (error out=w604:errorcluster)  [unwired: 1 in, 1 out]
                  }
                  frame True {
                  }
                }
              }
              frame "Set Temperature" {
                n225 = call "SetTemp_popup.vi"("error in (no error)"=w611) -> ("error out"=w616:errorcluster, "Cancel"=w609:bool, "Output Line Command"=w615:string)  [unwired: 7 in]
                n226 = Bundle By Name(cluster=w612, "Signal"=w609, "Command"=w615, "Add or modification"=TRUE) -> (w614:T2)
                n227 = case shown="True" w609 {
                  tunnel: w617 -> [w621 _]
                  tunnel: w616 -> [w620 w622]
                  tunnel: w614 -> [w619 _]
                  tunnel: [w618 w622] -> w613
                  frame False {
                    n228 = Generate User Event(user event=w621, event data cluster=w619, error in=w620) -> (error out=w618:errorcluster)  [unwired: 1 in, 1 out]
                  }
                  frame True {
                  }
                }
              }
              frame "Wait for Temperature" {
                n229 = call "SetWaitForTemp_popup.vi"("error in (no error)"=w625) -> ("Output Line Command"=w629:string, "Cancel"=w623:bool, "error out"=w630:errorcluster)  [unwired: 7 in]
                n230 = Bundle By Name(cluster=w626, "Signal"=w623, "Command"=w629, "Add or modification"=TRUE) -> (w628:T2)
                n231 = case shown="True" w623 {
                  tunnel: w631 -> [w635 _]
                  tunnel: w630 -> [w634 w636]
                  tunnel: w628 -> [w633 _]
                  tunnel: [w632 w636] -> w627
                  frame False {
                    n232 = Generate User Event(user event=w635, event data cluster=w633, error in=w634) -> (error out=w632:errorcluster)  [unwired: 1 in, 1 out]
                  }
                  frame True {
                  }
                }
              }
              frame "Wait for" {
                n233 = call "SetWaitFor_popup.vi"("error in (no error)"=w639) -> ("error out"=w644:errorcluster, "Cancel"=w637:bool, "Output Line Command"=w643:string)  [unwired: 7 in]
                n234 = Bundle By Name(cluster=w640, "Signal"=w637, "Command"=w643, "Add or modification"=TRUE) -> (w642:T2)
                n235 = case shown="False" w637 {
                  tunnel: w645 -> [w649 _]
                  tunnel: w644 -> [w648 w650]
                  tunnel: w642 -> [w647 _]
                  tunnel: [w646 w650] -> w641
                  frame False {
                    n236 = Generate User Event(user event=w649, event data cluster=w647, error in=w648) -> (error out=w646:errorcluster)  [unwired: 1 in, 1 out]
                  }
                  frame True {
                  }
                }
              }
              frame "Start" {
                n237 = call "SetStart_popup.vi"("error in (no error)"=w653) -> ("Output Line Command"=w657:string, "Cancel"=w651:bool, "error out"=w658:errorcluster)  [unwired: 7 in]
                n238 = Bundle By Name(cluster=w654, "Signal"=w651, "Command"=w657, "Add or modification"=TRUE) -> (w656:T2)
                n239 = case shown="True" w651 {
                  tunnel: w659 -> [w663 _]
                  tunnel: w658 -> [w662 w664]
                  tunnel: w656 -> [w661 _]
                  tunnel: [w660 w664] -> w655
                  frame False {
                    n240 = Generate User Event(user event=w663, event data cluster=w661, error in=w662) -> (error out=w660:errorcluster)  [unwired: 1 in, 1 out]
                  }
                  frame True {
                  }
                }
              }
              frame "Remarks" {
                n241 = call "SetRemarks_popup.vi"("error in (no error)"=w667) -> ("Cancel"=w665:bool, "Output Line Command"=w671:string, "error out"=w672:errorcluster)  [unwired: 7 in]
                n242 = Bundle By Name(cluster=w668, "Signal"=w665, "Command"=w671, "Add or modification"=TRUE) -> (w670:T2)
                n243 = case shown="True" w665 {
                  tunnel: w673 -> [w677 _]
                  tunnel: w672 -> [w676 w678]
                  tunnel: w670 -> [w675 _]
                  tunnel: [w674 w678] -> w669
                  frame False {
                    n244 = Generate User Event(user event=w677, event data cluster=w675, error in=w676) -> (error out=w674:errorcluster)  [unwired: 1 in, 1 out]
                  }
                  frame True {
                  }
                }
              }
              frame "Run Sequence" {
                n245 = call "SetRunSeq_popup.vi"("error in (no error)"=w681) -> ("error out"=w686:errorcluster, "Output Line Command"=w685:string, "Cancel"=w679:bool)  [unwired: 8 in]
                n246 = Bundle By Name(cluster=w682, "Signal"=w679, "Command"=w685, "Add or modification"=TRUE) -> (w684:T2)
                n247 = case shown="True" w679 {
                  tunnel: w687 -> [w691 _]
                  tunnel: w686 -> [w690 w692]
                  tunnel: w684 -> [w689 _]
                  tunnel: [w688 w692] -> w683
                  frame False {
                    n248 = Generate User Event(user event=w691, event data cluster=w689, error in=w690) -> (error out=w688:errorcluster)  [unwired: 1 in, 1 out]
                  }
                  frame True {
                  }
                }
              }
              frame "Run VI" {
                n249 = call "SetRunVI_popup.vi"("error in (no error)"=w695) -> ("Cancel"=w693:bool, "Output Line Command"=w699:string, "error out"=w700:errorcluster)  [unwired: 7 in]
                n250 = Bundle By Name(cluster=w696, "Signal"=w693, "Command"=w699, "Add or modification"=TRUE) -> (w698:T2)
                n251 = case shown="True" w693 {
                  tunnel: w701 -> [w705 _]
                  tunnel: w700 -> [w704 w706]
                  tunnel: w698 -> [w703 _]
                  tunnel: [w702 w706] -> w697
                  frame False {
                    n252 = Generate User Event(user event=w705, event data cluster=w703, error in=w704) -> (error out=w702:errorcluster)  [unwired: 1 in, 1 out]
                  }
                  frame True {
                  }
                }
              }
              frame "Abort VI" {
                n253 = call "SetAbortVI_popup.vi"("error in (no error)"=w709) -> ("Cancel"=w707:bool, "Output Line Command"=w713:string, "error out"=w714:errorcluster)  [unwired: 7 in]
                n254 = Bundle By Name(cluster=w710, "Signal"=w707, "Command"=w713, "Add or modification"=TRUE) -> (w712:T2)
                n255 = case shown="True" w707 {
                  tunnel: w715 -> [w719 _]
                  tunnel: w714 -> [w718 w720]
                  tunnel: w712 -> [w717 _]
                  tunnel: [w716 w720] -> w711
                  frame False {
                    n256 = Generate User Event(user event=w719, event data cluster=w717, error in=w718) -> (error out=w716:errorcluster)  [unwired: 1 in, 1 out]
                  }
                  frame True {
                  }
                }
              }
              frame "Set Parameter" {
                n257 = call "SetParameter_popup.vi"("error in (no error)"=w723) -> ("error out"=w728:errorcluster, "Cancel"=w721:bool, "Output Line Command"=w727:string)  [unwired: 7 in]
                n258 = Bundle By Name(cluster=w724, "Signal"=w721, "Command"=w727, "Add or modification"=TRUE) -> (w726:T2)
                n259 = case shown="False" w721 {
                  tunnel: w729 -> [w733 _]
                  tunnel: w728 -> [w732 w734]
                  tunnel: w726 -> [w731 _]
                  tunnel: [w730 w734] -> w725
                  frame False {
                    n260 = Generate User Event(user event=w733, event data cluster=w731, error in=w732) -> (error out=w730:errorcluster)  [unwired: 1 in, 1 out]
                  }
                  frame True {
                  }
                }
              }
              frame "Write to VISA instrument" {
                n261 = call "WriteVISA_popup.vi"("error in (no error)"=w737) -> ("Output Line Command"=w741:string, "Cancel"=w735:bool, "error out"=w742:errorcluster)  [unwired: 8 in]
                n262 = Bundle By Name(cluster=w738, "Signal"=w735, "Command"=w741, "Add or modification"=TRUE) -> (w740:T2)
                n263 = case shown="False" w735 {
                  tunnel: w743 -> [w747 _]
                  tunnel: w742 -> [w746 w748]
                  tunnel: w740 -> [w745 _]
                  tunnel: [w744 w748] -> w739
                  frame False {
                    n264 = Generate User Event(user event=w747, event data cluster=w745, error in=w746) -> (error out=w744:errorcluster)  [unwired: 1 in, 1 out]
                  }
                  frame True {
                  }
                }
              }
              frame "Set" {
                n265 = call "SetDevice_popup.vi"("error in (no error)"=w751) -> ("Cancel"=w749:bool, "Output Line Command"=w755:string, "error out"=w756:errorcluster)  [unwired: 7 in]
                n266 = Bundle By Name(cluster=w752, "Signal"=w749, "Command"=w755, "Add or modification"=TRUE) -> (w754:T2)
                n267 = case shown="True" w749 {
                  tunnel: w757 -> [w761 _]
                  tunnel: w756 -> [w760 w762]
                  tunnel: w754 -> [w759 _]
                  tunnel: [w758 w762] -> w753
                  frame False {
                    n268 = Generate User Event(user event=w761, event data cluster=w759, error in=w760) -> (error out=w758:errorcluster)  [unwired: 1 in, 1 out]
                  }
                  frame True {
                  }
                }
              }
              frame "Sweep" {
                n269 = call "SetDevice_popup.vi"("error in (no error)"=w765) -> ("Cancel"=w763:bool, "Output Line Command"=w769:string, "error out"=w770:errorcluster)  [unwired: 7 in]
                n270 = Bundle By Name(cluster=w766, "Signal"=w763, "Command"=w769, "Add or modification"=TRUE) -> (w768:T2)
                n271 = case shown="True" w763 {
                  tunnel: w771 -> [w775 _]
                  tunnel: w770 -> [w774 w776]
                  tunnel: w768 -> [w773 _]
                  tunnel: [w772 w776] -> w767
                  frame False {
                    n272 = Generate User Event(user event=w775, event data cluster=w773, error in=w774) -> (error out=w772:errorcluster)  [unwired: 1 in, 1 out]
                  }
                  frame True {
                  }
                }
              }
              frame "Stop" {
                w777 = FALSE ("Signal")
                n273 = Bundle By Name(cluster=w781, "Signal"=w777, "Command"="Stop", "Add or modification"=TRUE) -> (w783:T2)
                n274 = case shown="False" w777 {
                  tunnel: w784 -> [w788 _]
                  tunnel: w783 -> [w787 _]
                  tunnel: [w786 w789] -> w782
                  tunnel: w778 -> [w785 w789]
                  frame False {
                    n275 = Generate User Event(user event=w788, event data cluster=w787, error in=w785) -> (error out=w786:errorcluster)  [unwired: 1 in, 1 out]
                  }
                  frame True {
                  }
                }
              }
              frame "Wait for Field Stable" {
                w790 = FALSE ("Signal")
                n276 = Bundle By Name(cluster=w795, "Signal"=w790, "Command"="Wait for Field Stable", "Add or modification"=TRUE) -> (w791:T2)
                n277 = case shown="True" w790 {
                  tunnel: w797 -> [w801 _]
                  tunnel: w791 -> [w800 _]
                  tunnel: [w799 w802] -> w796
                  tunnel: w792 -> [w798 w802]
                  frame False {
                    n278 = Generate User Event(user event=w801, event data cluster=w800, error in=w798) -> (error out=w799:errorcluster)  [unwired: 1 in, 1 out]
                  }
                  frame True {
                  }
                }
              }
              frame "Wait for VI value" {
                n279 = call "SetWaitForAnyVI_popup.vi"("error in (no error)"=w807) -> ("error out"=w803:errorcluster, "Cancel"=w804:bool, "Output Line Command"=w806:string)  [unwired: 7 in]
                n280 = Bundle By Name(cluster=w809, "Signal"=w804, "Command"=w806, "Add or modification"=TRUE ("Signal")) -> (w808:T2)
                n281 = case shown="False" w804 {
                  tunnel: w811 -> [w815 _]
                  tunnel: w808 -> [w814 _]
                  tunnel: [w813 w816] -> w810
                  tunnel: w803 -> [w812 w816]
                  frame False {
                    n282 = Generate User Event(user event=w815, event data cluster=w814, error in=w812) -> (error out=w813:errorcluster)  [unwired: 1 in, 1 out]
                  }
                  frame True {
                  }
                }
              }
              frame "Run Macro" {
                n283 = call "RunMacro_popup.vi"("load?"=FALSE, "error in (no error)"=w822) -> ("Cancel"=w819:bool, "command out"=w817:string, "error out"=w820:errorcluster)  [unwired: 6 in]
                n284 = Bundle By Name(cluster=w824, "Signal"=w819, "Command"=w817, "Add or modification"=TRUE ("Signal")) -> (w823:T2)
                n285 = case shown="False" w819 {
                  tunnel: w826 -> [w830 _]
                  tunnel: w823 -> [w829 _]
                  tunnel: [w828 w831] -> w825
                  tunnel: w820 -> [w827 w831]
                  frame False {
                    n286 = Generate User Event(user event=w830, event data cluster=w829, error in=w827) -> (error out=w828:errorcluster)  [unwired: 1 in, 1 out]
                  }
                  frame True {
                  }
                }
              }
            }
          }
          event "Sequence": Double Click {
            # "check if the sequence is changed.\n(1) 'cancel' button pressed \nOR (2) no value is changed"
            n287 = event-data() -> ("Row"=w844:i32)  [unwired: 1 in]
            n288 = Unbundle By Name(w843) -> ("Sequence Reference"=w848:refnum<vi>)
            n289 = Bundle By Name(cluster=w853, "No. of line"=w844) -> (w852:T1)
            n290 = call "Library2.vi"("Message_command_in"=w852, "error in (no error)"=w851) -> ("Message_command out"=w850:T3, "error out"=w847:errorcluster)  [unwired: 7 in]
            n291 = Unbundle By Name(w850) -> ("No. of command"=w849:i32)
            n292 = property class="LstBox (strict)"(reference=w848, error in=w847) -> (error out=w846:errorcluster, "Item Names"=w845:string[])  [unwired: 1 out]
            n293 = Index Array(array=w845, index=w844) -> (element=w836:string)
            n294 = case shown="15" w849 {
              tunnel: w846 -> [w869 w876 w883 w890 w897 w903 w912 w919 w926 w933 w940 w947 w954 w961 w965]
              tunnel: w836 -> [w868 w875 w882 w889 w896 w901 w911 w918 w925 w932 w939 w946 w953 w960 _]
              tunnel: w843 -> [w866 w873 w880 w887 w894 w905 w909 w916 w923 w930 w937 w944 w951 w957 w964]
              tunnel: w842 -> [w865 w872 w879 w886 w893 w904 w908 w915 w922 w929 w936 w943 w950 w956 w963]
              tunnel: [w867 w874 w881 w888 w895 w902 w910 w917 w924 w931 w938 w945 w952 w958 w965] -> w839
              tunnel: [w866 w873 w880 w887 w894 w905 w909 w916 w923 w930 w937 w944 w951 w957 w964] -> w841
              tunnel: [w865 w872 w879 w886 w893 w904 w908 w915 w922 w929 w936 w943 w950 w956 w963] -> w840
              tunnel: [w864 w871 w878 w885 w892 w899 w907 w914 w921 w928 w934 w941 w948 w955 TRUE ("Cancel")] -> w833
              tunnel: [w863 w870 w877 w884 w891 w898 w906 w913 w920 w927 w935 w942 w949 w959 _] -> w835
              frame 0 {
                n295 = call "SetField_popup.vi"("error in (no error)"=w869, "Input Line command"=w868) -> ("Output Line command"=w863:string, "Cancel"=w864:bool, "error out"=w867:errorcluster)  [unwired: 4 in]
              }
              frame 1 {
                n296 = call "SetTemp_popup.vi"("Input Line Command"=w875, "error in (no error)"=w876) -> ("error out"=w874:errorcluster, "Cancel"=w871:bool, "Output Line Command"=w870:string)  [unwired: 6 in]
              }
              frame 2 {
                n297 = call "SetStart_popup.vi"("Input Line Command"=w882, "error in (no error)"=w883) -> ("Output Line Command"=w877:string, "Cancel"=w878:bool, "error out"=w881:errorcluster)  [unwired: 6 in]
              }
              frame 4 {
                n298 = call "SetWaitForTemp_popup.vi"("Input Line Command"=w889, "error in (no error)"=w890) -> ("Output Line Command"=w884:string, "Cancel"=w885:bool, "error out"=w888:errorcluster)  [unwired: 6 in]
              }
              frame 7 {
                n299 = call "SetRemarks_popup.vi"("Input Line Command"=w896, "error in (no error)"=w897) -> ("Cancel"=w892:bool, "Output Line Command"=w891:string, "error out"=w895:errorcluster)  [unwired: 6 in]
              }
              frame 8 {
                n300 = call "RunMacro_popup.vi"("load?"=TRUE, "command in"=w901, "error in (no error)"=w903) -> ("Cancel"=w899:bool, "command out"=w898:string, "error out"=w902:errorcluster)  [unwired: 5 in]
              }
              frame 9 {
                n301 = call "SetRunVI_popup.vi"("Input Line Command"=w911, "error in (no error)"=w912) -> ("Cancel"=w907:bool, "Output Line Command"=w906:string, "error out"=w910:errorcluster)  [unwired: 6 in]
              }
              frame 10 {
                n302 = call "SetAbortVI_popup.vi"("Input Line Command"=w918, "error in (no error)"=w919) -> ("Cancel"=w914:bool, "Output Line Command"=w913:string, "error out"=w917:errorcluster)  [unwired: 6 in]
              }
              frame 11 {
                n303 = call "SetDevice_popup.vi"("Input Line Command"=w925, "error in (no error)"=w926) -> ("Cancel"=w921:bool, "Output Line Command"=w920:string, "error out"=w924:errorcluster)  [unwired: 6 in]
              }
              frame 16 {
                n304 = call "SetSweep_popup.vi"("Input Line Command"=w932, "error in (no error)"=w933) -> ("Cancel"=w928:bool, "Output Line Command"=w927:string, "error out"=w931:errorcluster)  [unwired: 6 in]
              }
              frame 12 {
                n305 = call "SetWaitFor_popup.vi"("Input Line Command"=w939, "error in (no error)"=w940) -> ("error out"=w938:errorcluster, "Cancel"=w934:bool, "Output Line Command"=w935:string)  [unwired: 6 in]
              }
              frame 13 {
                n306 = call "SetParameter_popup.vi"("Input Line Command"=w946, "error in (no error)"=w947) -> ("error out"=w945:errorcluster, "Cancel"=w941:bool, "Output Line Command"=w942:string)  [unwired: 6 in]
              }
              frame 15 {
                n307 = call "WriteVISA_popup.vi"("error in (no error)"=w954, "Input Line Command"=w953) -> ("Output Line Command"=w949:string, "Cancel"=w948:bool, "error out"=w952:errorcluster)  [unwired: 7 in]
              }
              frame 14 {
                n308 = call "SetWaitForAnyVI_popup.vi"("Input Line Command"=w960, "error in (no error)"=w961) -> ("error out"=w958:errorcluster, "Cancel"=w955:bool, "Output Line Command"=w959:string)  [unwired: 6 in]
              }
              frame Default {
              }
            }
            n309 = Equal?(x=w836, y=w835) -> (x = y?=w834:bool)
            n310 = Or(x=w833, y=w834) -> (x .or. y?=w832:bool)
            n311 = case shown="False" w832 {
              selector: w832 -> [w856 _]
              tunnel: w841 -> [w860 _]
              tunnel: w840 -> [w858 _]
              tunnel: w835 -> [w857 _]
              tunnel: w839 -> [w855 w862]
              tunnel: [w854 w862] -> w838
              frame False {
                n312 = Bundle By Name(cluster=w860, "Signal"=w856, "Command"=w857, "Add or modification"=FALSE) -> (w859:T2)
                n313 = Generate User Event(user event=w858, event data cluster=w859, error in=w855) -> (error out=w854:errorcluster)  [unwired: 1 in, 1 out]
              }
              frame True {
              }
            }
          }
          event "Sequence": Value Change {
            n314 = event-data() -> ("NewVal"=w970:i32[])  [unwired: 1 in]
            n315 = Index Array(array=w970, index=0) -> (element=→"Cursor Position":i32)
          }
          event "cancel", "accept/return": Value Change {
            # "Press OK button saves the sequence and exit"
            n316 = event-data() -> ("CtlRef"=w974:refnum<vi>)  [unwired: 1 in, 5 out]
            n317 = property class="Bool"(reference=w974) -> ("Label.Text"=w973:string)  [unwired: 1 in, 2 out]
            n318 = Equal?(x=w973, y="cancel") -> (x = y?=w971:bool)
            "do not update seq." <- w971
            n319 = case shown="False" w971 {
              frame False {
                n320 = property on="Sequence" class="LstBox (strict)"() -> ("Item Names"=→"changed sequence":string[])  [unwired: 2 in, 2 out]
              }
              frame True {
              }
            }
          }
        }
      }
    }
    frame Error {
    }
  }
  n321 = Unregister For Events(event registration refnum=w22, error in=w21) -> (error out=→"error out":errorcluster)
  "Buffer History" <- w15
  "Buffer Edit" <- w15
